vi "Facade.vi"(0 "Data In":T4, 2 "Display State In":T2, 3 "Container State":T3) -> (6 "Data Out":T4, 7 "Display State Out":T2, 8 "Action":T1)   [LabVIEW 2019, in "XControlShutter.xctl"]
uses:
  XControlShutter.xctl
  Data.ctl
  <vilib>/_xctls/Container State.ctl
  State.ctl
  <vilib>/_xctls/Action.ctl
  <vilib>/_xctls/XControlSupport.lvlib
panel:
  in  "399button":bool
  out "399cover":bool
  in  "935button":bool
  out "935cover":bool
  in  "369button":bool
  out "369cover":bool
  in  "All off":bool
  in  "All on":bool
  # "399"
  # "369"
  # "935"
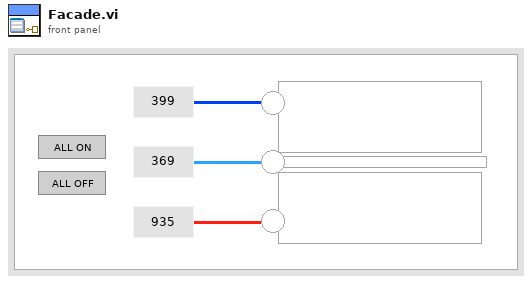
[diagram p1: front panel]
types:
  T1 = typedef "XControlSupport.lvlib/Action.ctl" = cluster{"Data Changed?":bool, "State Changed?":bool, "Action Name":string}
  T2 = typedef "XControlShutter.xctl/State.ctl" = cluster{"Numeric":dbl}
  T3 = typedef "XControlSupport.lvlib/Container State.ctl" = cluster{"Indicator?":bool, "Run Mode?":bool, " Refnum":refnum<vi>}
  T4 = typedef "XControlShutter.xctl/Data.ctl" = dbl
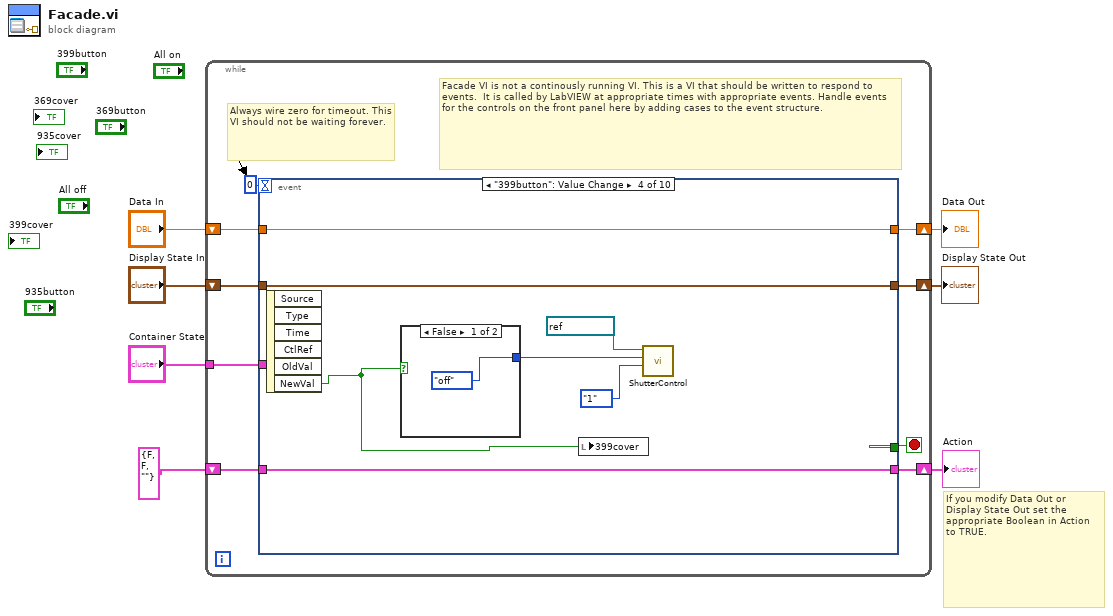
[diagram p0: block diagram]
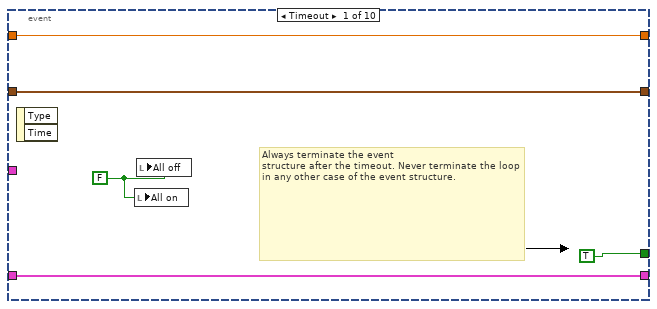
[diagram p2: hidden frame]
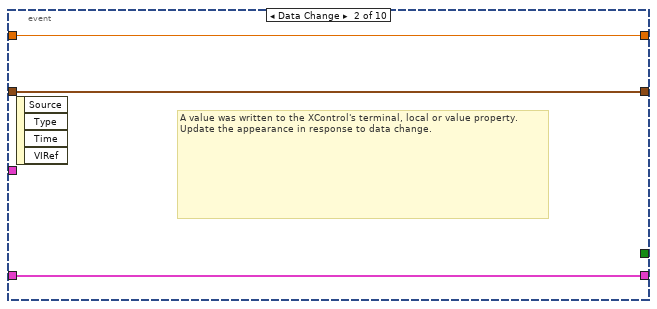
[diagram p3: hidden frame]
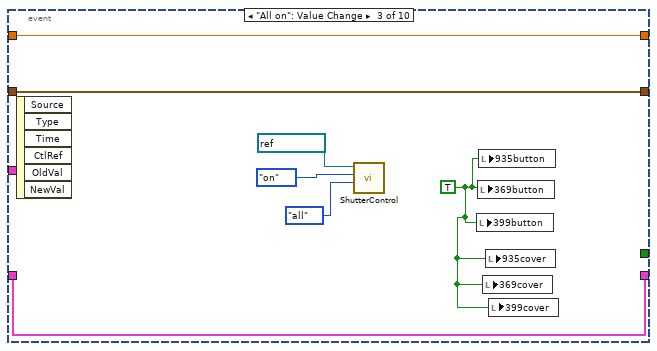
[diagram p4: hidden frame]
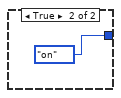
[diagram p5: hidden frame]
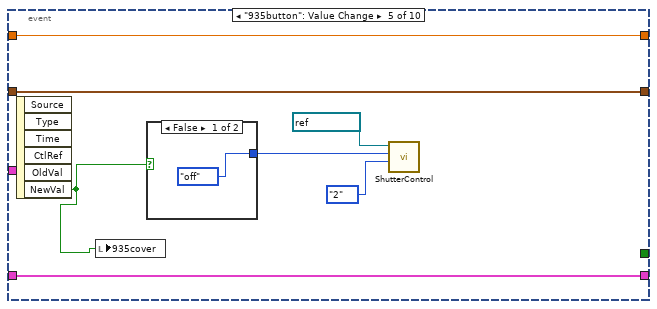
[diagram p6: hidden frame]
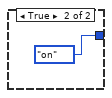
[diagram p7: hidden frame]
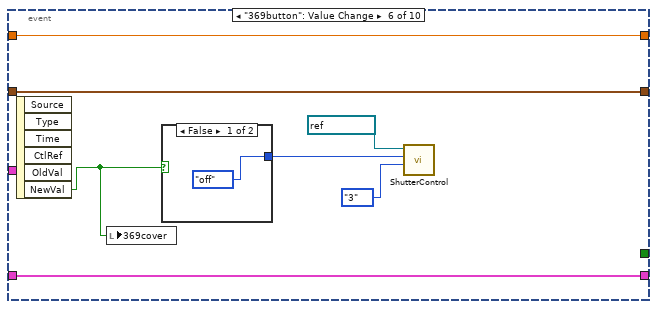
[diagram p8: hidden frame]
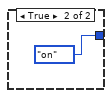
[diagram p9: hidden frame]
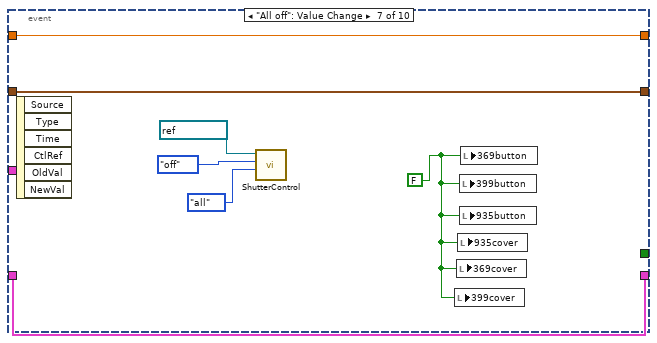
[diagram p10: hidden frame]
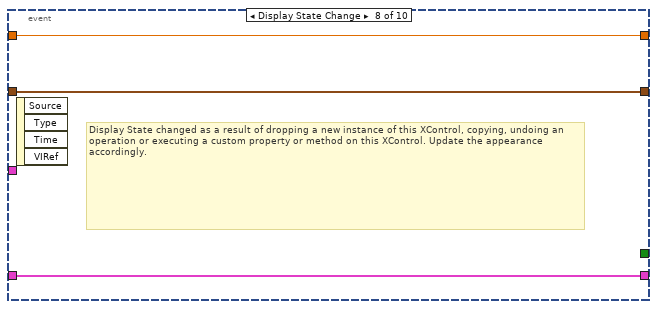
[diagram p11: hidden frame]
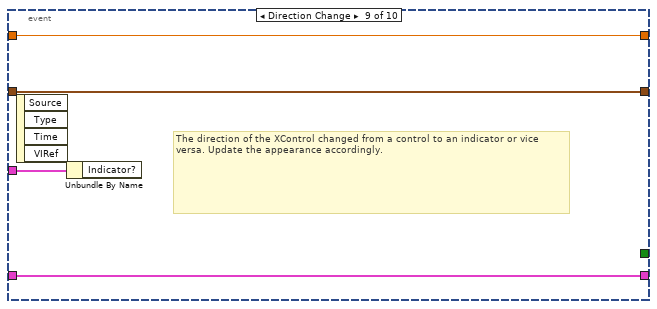
[diagram p12: hidden frame]
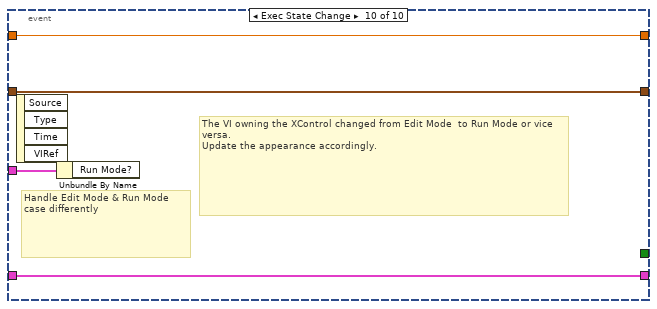
[diagram p13: hidden frame]
diagram:
  # "If you modify Data Out or\nDisplay State Out set the\nappropriate Boolean in Action\nto TRUE."
  n1 = while {
    shift-right: [w15] -> w4
    shift-left: "Display State In" -> [w16]
    tunnel: "Container State" -> [w12]
    shift-right: [w10] -> w7
    shift-left: "Data In" -> [w11]
    shift-right: [w8] -> w2
    shift-left: T1 {"Data Changed?"=FALSE, "State Changed?"=FALSE, "Action Name"=""} ("Action") -> [w9]
    stop <- w14 stop-if-true
    # "Facade VI is not a continously running VI. This is a VI that should be written to respond to events.  It is called by LabVIEW at appropriate times with appropriate events. Handle events for the controls on the front panel here by adding cases to the event structure."
    # "Always wire zero for timeout. This\nVI should not be waiting forever."
    n2 = event shown="[3] \"399button\": Value Change" {
      selector: _ -> [_ _ _ _ _ _ _ _ _ _]
      dyn-events: _ -> [_ _ _ _ _ _ _ _ _ _]
      timeout: 0 -> [_ _ _ _ _ _ _ _ _ _]
      tunnel: w16 -> [w19 w23 w31 w38 w47 w56 w65 w68 w71 w75]
      tunnel: [w19 w23 w31 w38 w47 w56 w65 w68 w71 w75] -> w15
      tunnel: [TRUE _ _ _ _ _ _ _ _ _] -> w14
      tunnel: w12 -> [_ _ _ _ _ _ _ _ w72 w76]
      tunnel: w11 -> [w18 w24 w30 w37 w46 w55 w64 w67 w70 w74]
      tunnel: [w18 w24 w30 w37 w46 w55 w64 w67 w70 w74] -> w10
      tunnel: [w20 w22 w29 w36 w45 w54 w63 w66 w69 w73] -> w8
      tunnel: w9 -> [w20 w22 w29 w36 w45 w54 w63 w66 w69 w73]
      event Timeout {
        w17 = FALSE
        # "Always terminate the event\nstructure after the timeout. Never terminate the loop in any other case of the event structure."
        n3 = event-data() -> ()  [unwired: 1 in, 2 out]
        n4 = local write "All on"(w17) -> ()
        n5 = local write "All off"(w17) -> ()
      }
      event Data Change {
        # "A value was written to the XControl's terminal, local or value property.\nUpdate the appearance in response to data change."
        n6 = event-data() -> ()  [unwired: 1 in, 4 out]
      }
      event "All on": Value Change {
        w25 = TRUE
        n7 = event-data() -> ()  [unwired: 1 in, 6 out]
        n8 = call "ShutterControl.vi"("id"=enum16{"1", "2", "3", "4", "all"}."all", "cmd"=enum16{"off", "on"}."on", "VISA resource name"=refnum<visa-resource-name> "COM11") -> ()  [unwired: 8 in, 1 out]
        n9 = local write "399button"(w25) -> ()
        n10 = local write "369button"(w25) -> ()
        n11 = local write "935button"(w25) -> ()
        n12 = local write "369cover"(w25) -> ()
        n13 = local write "935cover"(w25) -> ()
        n14 = local write "399cover"(w25) -> ()
      }
      event "399button": Value Change {
        n15 = event-data() -> ("NewVal"=w32:bool)  [unwired: 1 in, 5 out]
        n16 = case shown="False" w32 {
          tunnel: [enum16{"off", "on"}."off" ("cmd") enum16{"off", "on"}."on" ("cmd")] -> w33
          frame False {
          }
          frame True {
          }
        }
        n17 = local write "399cover"(w32) -> ()
        n18 = call "ShutterControl.vi"("id"=enum16{"1", "2", "3", "4", "all"}."1", "cmd"=w33, "VISA resource name"=refnum<visa-resource-name> "COM11") -> ()  [unwired: 8 in, 1 out]
      }
      event "935button": Value Change {
        n19 = event-data() -> ("NewVal"=w41:bool)  [unwired: 1 in, 5 out]
        n20 = local write "935cover"(w41) -> ()
        n21 = case shown="False" w41 {
          tunnel: [enum16{"off", "on"}."off" ("cmd") enum16{"off", "on"}."on" ("cmd")] -> w42
          frame False {
          }
          frame True {
          }
        }
        n22 = call "ShutterControl.vi"("id"=enum16{"1", "2", "3", "4", "all"}."2", "cmd"=w42, "VISA resource name"=refnum<visa-resource-name> "COM11") -> ()  [unwired: 8 in, 1 out]
      }
      event "369button": Value Change {
        n23 = event-data() -> ("NewVal"=w50:bool)  [unwired: 1 in, 5 out]
        n24 = local write "369cover"(w50) -> ()
        n25 = case shown="False" w50 {
          tunnel: [enum16{"off", "on"}."off" ("cmd") enum16{"off", "on"}."on" ("cmd")] -> w51
          frame False {
          }
          frame True {
          }
        }
        n26 = call "ShutterControl.vi"("id"=enum16{"1", "2", "3", "4", "all"}."3", "cmd"=w51, "VISA resource name"=refnum<visa-resource-name> "COM11") -> ()  [unwired: 8 in, 1 out]
      }
      event "All off": Value Change {
        w59 = FALSE
        n27 = event-data() -> ()  [unwired: 1 in, 6 out]
        n28 = call "ShutterControl.vi"("id"=enum16{"1", "2", "3", "4", "all"}."all", "cmd"=enum16{"off", "on"}."off", "VISA resource name"=refnum<visa-resource-name> "COM11") -> ()  [unwired: 8 in, 1 out]
        n29 = local write "399cover"(w59) -> ()
        n30 = local write "369cover"(w59) -> ()
        n31 = local write "935cover"(w59) -> ()
        n32 = local write "399button"(w59) -> ()
        n33 = local write "935button"(w59) -> ()
        n34 = local write "369button"(w59) -> ()
      }
      event Display State Change {
        # "Display State changed as a result of dropping a new instance of this XControl, copying, undoing an operation or executing a custom property or method on this XControl. Update the appearance accordingly."
        n35 = event-data() -> ()  [unwired: 1 in, 4 out]
      }
      event Direction Change {
        # "The direction of the XControl changed from a control to an indicator or vice versa. Update the appearance accordingly."
        n36 = event-data() -> ()  [unwired: 1 in, 4 out]
        n37 = Unbundle By Name(w72) -> ()  [unwired: 1 out]
      }
      event Exec State Change {
        # "The VI owning the XControl changed from Edit Mode  to Run Mode or vice versa.\nUpdate the appearance accordingly."
        # "Handle Edit Mode & Run Mode\ncase differently"
        n38 = event-data() -> ()  [unwired: 1 in, 4 out]
        n39 = Unbundle By Name(w76) -> ()  [unwired: 1 out]
      }
    }
  }
  "Display State Out" <- w4
  "Data Out" <- w7
  "Action" <- w2
